vi "生成XY图.vi"(3 "堆叠数据":bool, 4 "测试数据":dbl[][](array[numeric]), 5 "功能选择":enum16{"扫描", "测试中", "刷新"}(ring), 6 "曲线设置":T1={"X轴数据选择"=enum."设置电压", "Y轴组"=[]}, 8 "错误输入（无错误）":errorcluster, 11 "XY图":refnum<vi>) -> (0 "错误输出":errorcluster)   [LabVIEW 2021]
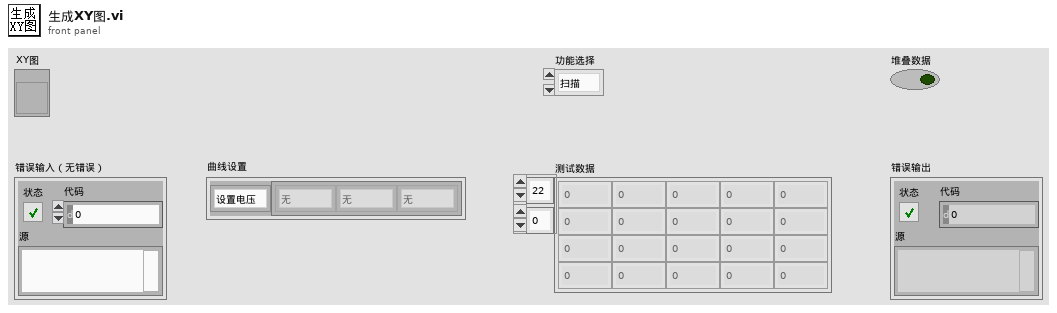
[diagram p1: front panel]
types:
  T1 = typedef "曲线设置.ctl" = cluster{"X轴数据选择":enum16{"时间", "设置电压", "读取电流", "读取电压"}, "Y轴组":enum16{"时间", "设置电压", "读取电流", "读取电压", "无"}[]}
  T2 = cluster{"Name":string, "Color":u32, "Style":u8, "Point Style":u8, "Name Visible":bool, "Allow Drag":bool, "Cursor Mode":u32, "Plot":i32, "Index":i32, "Position":cluster{"X":dbl, "Y":dbl}, "X Scale":u32, "Y Scale":u32, "Watch Plots":i32[], "Watch All Plots":bool, "Plot Area":i32, "Label Offset":cluster{"X":i32, "Y":i32}}
  T3 = typedef "曲线属性.ctl" = cluster{"曲线名":string, "曲线颜色":u32}[]
  T4 = cluster{"Name":string, "Color":u32, "Style":u8, "Point Style":u8, "Name Visible":bool, "Allow Drag":bool, "Cursor Mode":u32, "Plot":i32, "Index":i32, "Position":cluster{"X":dbl, "Y":dbl}, "X Scale":u32, "Y Scale":u32, "Watch Plots":i32[], "Watch All Plots":bool, "Plot Area":i32, "Label Offset":cluster{"X":i32, "Y":i32}}[]
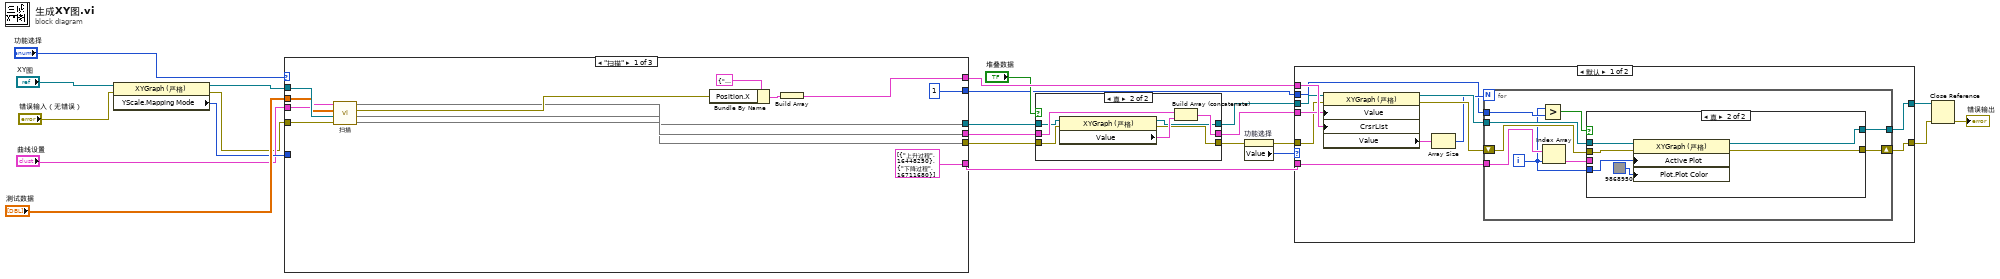
[diagram p0: block diagram]
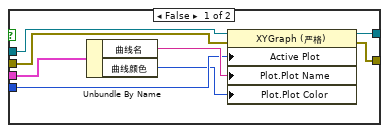
[diagram p2: hidden frame]
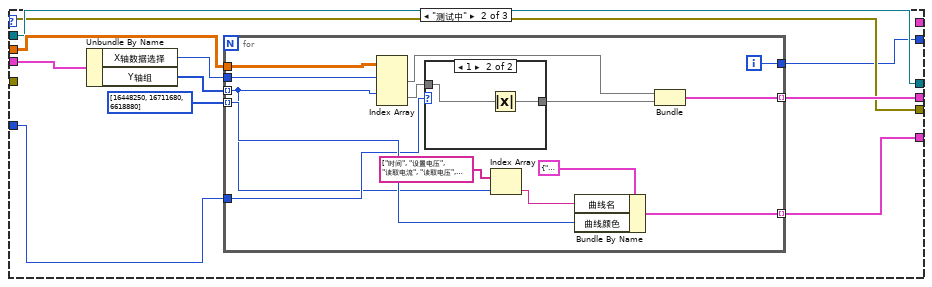
[diagram p5: hidden frame]
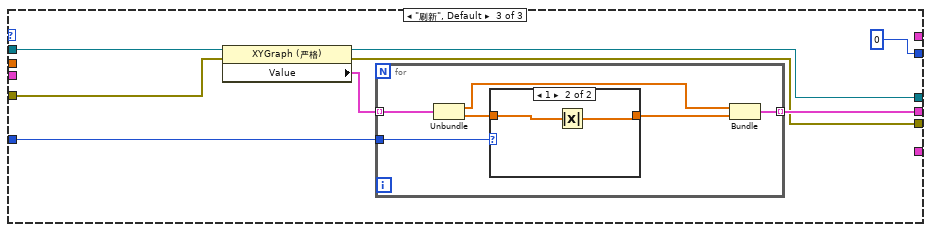
[diagram p7: hidden frame]
diagram:
  n1 = property class="XYGraph (严格)"(reference="XY图", error in="错误输入（无错误）") -> (reference out=w9:refnum<vi>, error out=w8:errorcluster, "YScale.Mapping Mode"=w11:u8)
  n2 = case shown="\"扫描\"" "功能选择" {
    tunnel: "测试数据" -> [w29 w47 _]
    tunnel: [w26 w46 w69] -> w17
    tunnel: [w36 _ _] -> w18
    tunnel: [T3 [{"曲线名"="上升过程", "曲线颜色"=16448250}, {"曲线名"="下降过程", "曲线颜色"=16711680}] ("曲线属性") w44 _] -> w14
    tunnel: w11 -> [_ w43 w68]
    tunnel: "曲线设置" -> [w28 w42 _]
    tunnel: w9 -> [w31 w39 w72]
    tunnel: w8 -> [w30 w38 w71]
    tunnel: [w25 w39 w67] -> w7
    tunnel: [w24 w38 w66] -> w6
    tunnel: [1 w37 0] -> w1
    frame "扫描" {
      n3 = call "扫描.vi"("曲线设置"=w30, 9:w31, "错误输入（无错误）"=w29, 11:w28) -> (0:w24, 1:w25, "错误输出"=w27:errorcluster, 3:w26)  [unwired: 4 in]
      n4 = Bundle By Name(cluster=T2 {"Name"="游标", "Color"=16776960, "Style"=2, "Point Style"=13, "Name Visible"=FALSE, "Allow Drag"=TRUE, "Cursor Mode"=2, "Plot"=-1, "Index"=0, "Position"={"X"=0.0, "Y"=0.0}, "X Scale"=0, "Y Scale"=0, "Watch Plots"=[], "Watch All Plots"=TRUE, "Plot Area"=0, "Label Offset"={"X"=0, "Y"=0}}, "Position.X"=w27) -> (w33:T2)
      n5 = Build Array(w33) -> (w36:T4)
    }
    frame "测试中" {
      n6 = Unbundle By Name(w42) -> ("X轴数据选择"=w41:enum16{"时间", "设置电压", "读取电流", "读取电压"}, "Y轴组"=w40:enum16{"时间", "设置电压", "读取电流", "读取电压", "无"}[])
      n7 = for {
        tunnel: w40 -> [w51] mode=indexing
        tunnel: w47 -> [w61]
        tunnel: [w59] -> w46 mode=indexing
        tunnel: w41 -> [w58]
        tunnel: u32[] [16448250, 16711680, 6618880] -> [w57] mode=indexing
        tunnel: [w56] -> w44 mode=indexing
        tunnel: w43 -> [w55]
        tunnel: [w48] -> w37
        i -> [w48]
        n8 = Index Array(array=w61, index (row) #1=w58, index (row) #2=w51) -> (element #1=w60:dbl[], element #2=w54:dbl[])  [unwired: 2 in]
        n9 = case shown="1" w55 {
          tunnel: w54 -> [w62 w64]
          tunnel: [w62 w63] -> w53
          frame 0, Default {
          }
          frame 1 {
            n10 = Absolute Value(x=w64) -> (abs(x)=w63:dbl[])
          }
        }
        n11 = Index Array(array=string[] ["时间", "设置电压", "读取电流", "读取电压", "无"] ("字符串[]"), index=w51) -> (element=w50:string)
        n12 = Bundle By Name(cluster=cluster{"曲线名":string, "曲线颜色":u32} {"曲线名"="0", "曲线颜色"=0}, "曲线名"=w50, "曲线颜色"=w57) -> (w56:cluster{"曲线名":string, "曲线颜色":u32})
        n13 = Bundle("测试数据"=w60, "测试数据"=w53) -> (w59:cluster{"测试数据":dbl[], "测试数据":dbl[]})  [unwired: 1 in]
      }
    }
    frame "刷新", Default {
      n14 = property class="XYGraph (严格)"(reference=w72, error in=w71) -> (reference out=w67:refnum<vi>, error out=w66:errorcluster, "Value"=w70:cluster{"测试数据":dbl[], "测试数据":dbl[]}[])
      n15 = for {
        tunnel: w70 -> [w78] mode=indexing
        tunnel: w68 -> [w77]
        tunnel: [w73] -> w69 mode=indexing
        n16 = Unbundle(w78) -> ("测试数据"=w74:dbl[], "测试数据"=w76:dbl[])
        n17 = case shown="1" w77 {
          tunnel: w76 -> [w79 w81]
          tunnel: [w79 w80] -> w75
          frame 0, Default {
          }
          frame 1 {
            n18 = Absolute Value(x=w81) -> (abs(x)=w80:dbl[])
          }
        }
        n19 = Bundle("测试数据"=w74, "测试数据"=w75) -> (w73:cluster{"测试数据":dbl[], "测试数据":dbl[]})  [unwired: 1 in]
      }
    }
  }
  n20 = case shown="真" "堆叠数据" {
    tunnel: w17 -> [w84 w91]
    tunnel: [w84 w89] -> w16
    tunnel: [w82 w88] -> w15
    tunnel: [w83 w87] -> w4
    tunnel: w7 -> [w82 w86]
    tunnel: w6 -> [w83 w85]
    frame False {
    }
    frame True {
      n21 = property class="XYGraph (严格)"(reference=w86, error in=w85) -> (reference out=w88:refnum<vi>, error out=w87:errorcluster, "Value"=w90:cluster{"测试数据":dbl[], "测试数据":dbl[]}[])
      n22 = Build Array (concatenate)(w91, w90) -> (w89:cluster{"测试数据":dbl[], "测试数据":dbl[]}[])
    }
  }
  n23 = property on="功能选择" class="Enum (严格)"(error in=w4) -> (error out=w3:errorcluster, "Value"=w5:enum16{"扫描", "测试中", "刷新"})  [unwired: 1 in, 1 out]
  n24 = case shown="默认" w5 {
    tunnel: [w103 w128] -> w20
    tunnel: [w102 w127] -> w19
    tunnel: w18 -> [w101 _]
    tunnel: w16 -> [w100 _]
    tunnel: w15 -> [w99 w128]
    tunnel: w3 -> [w98 w127]
    tunnel: w14 -> [w97 _]
    tunnel: w1 -> [w92 _]
    frame Default {
      n25 = property class="XYGraph (严格)"(reference=w99, error in=w98, "Value"=w100, "CrsrList"=w101) -> (reference out=w96:refnum<vi>, error out=w95:errorcluster, "Value"=w94:cluster{"测试数据":dbl[], "测试数据":dbl[]}[])
      n26 = Array Size(array=w94) -> (size(s)=w93:i32)
      n27 = for {
        N: w93 -> [_]
        shift-right: [w111] -> w102
        shift-left: w95 -> [w112]
        tunnel: w97 -> [w106]
        tunnel: w96 -> [w110]
        tunnel: [w109] -> w103
        tunnel: w92 -> [w108]
        i -> [w105]
        n28 = Greater?(x=w105, y=w108) -> (0:w107:bool)
        n29 = Index Array(array=w106, index=w105) -> (element=w104:cluster{"曲线名":string, "曲线颜色":u32})
        n30 = case shown="真" w107 {
          tunnel: w112 -> [w119 w125]
          tunnel: [w118 w121] -> w111
          tunnel: w104 -> [w117 _]
          tunnel: w110 -> [w116 w126]
          tunnel: [w115 w122] -> w109
          tunnel: w105 -> [w114 w124]
          frame False {
            n31 = Unbundle By Name(w117) -> ("曲线名"=w120:string, "曲线颜色"=w113:u32)
            n32 = property on="属性节点" class="XYGraph (严格)"(reference=w116, error in=w119, "Active Plot"=w114, "Plot.Plot Name"=w120, "Plot.Plot Color"=w113) -> (reference out=w115:refnum<vi>, error out=w118:errorcluster)
          }
          frame True {
            n33 = property on="属性节点" class="XYGraph (严格)"(reference=w126, error in=w125, "Active Plot"=w124, "Plot.Plot Color"=u32 9868950 ("曲线.曲线颜色")) -> (reference out=w122:refnum<vi>, error out=w121:errorcluster)
          }
        }
      }
    }
    frame "刷新" {
    }
  }
  n34 = Close Reference(reference=w20, error in (no error)=w19) -> (error out=→"错误输出":errorcluster)
